vi "Add Timestamps to Rx Channels.vi"(8 "error in":errorcluster, 9 "timestamps":T1[](array[typedef]) format="%.0x", 10 "RxBC channel handles":T1[](array[typedef]) format="%.0x", 11 "RxRT channel handles":T1[](array[typedef]) format="%.0x") -> (0 "error out":errorcluster, 3 "Rx channel handles":T1[](array[typedef]) format="%.0x")   [LabVIEW 2020, in "Ballard MIL-STD-1553 Engine.lvlib" / "Implementation.lvlib" / "Execution Unit.lvclass"]
uses:
  Execution Unit.lvclass
  <vilib>/NI VeriStand/Custom Device API/Custom Device Item Ref.ctl
  <vilib>/NI VeriStand/Custom Device API/Custom Device API.lvlib
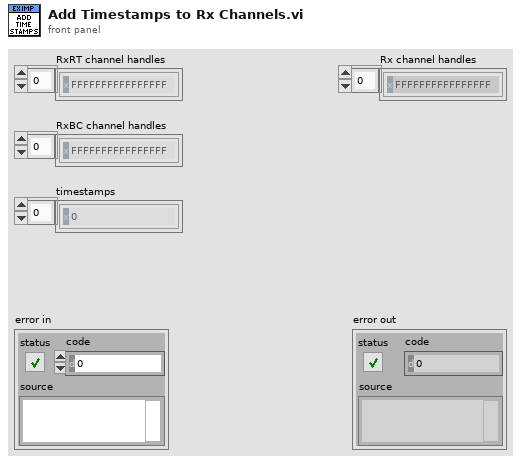
[diagram p1: front panel]
types:
  T1 = typedef "Custom Device API.lvlib/Custom Device Item Ref.ctl" = u64
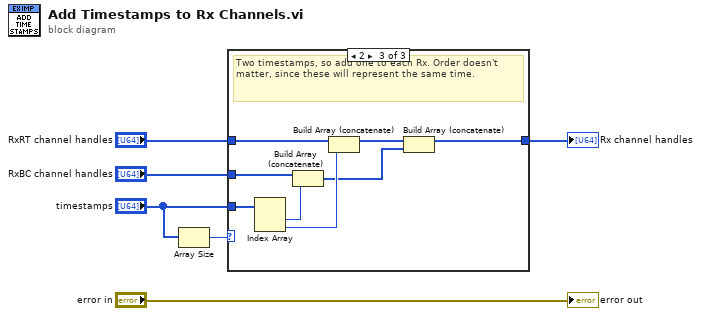
[diagram p0: block diagram]
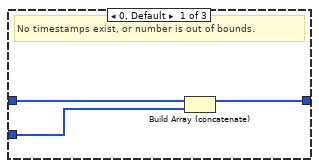
[diagram p2: hidden frame]
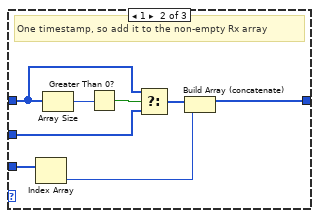
[diagram p3: hidden frame]
diagram:
  n1 = Array Size(array="timestamps") -> (size(s)=w5:i32)
  n2 = case shown="2" w5 {
    tunnel: "RxRT channel handles" -> [w9 w15 w22]
    tunnel: "RxBC channel handles" -> [w8 w14 w24]
    tunnel: [w7 w10 w18] -> w2
    tunnel: "timestamps" -> [_ w12 w25]
    frame 0, Default {
      # "No timestamps exist, or number is out of bounds."
      n3 = Build Array (concatenate)(w9, w8) -> (w7:T1[])
    }
    frame 1 {
      # "One timestamp, so add it to the non-empty Rx array"
      n4 = Index Array(array=w12) -> (element=w11:T1)  [unwired: 1 in]
      n5 = Array Size(array=w15) -> (size(s)=w17:i32)
      n6 = Greater Than 0?(x=w17) -> (x > 0?=w16:bool)
      n7 = Select(t=w15, s=w16, f=w14) -> (s? t:f=w13:T1[])
      n8 = Build Array (concatenate)(w13, w11) -> (w10:T1[])
    }
    frame 2 {
      # "Two timestamps, so add one to each Rx. Order doesn't matter, since these will represent the same time."
      n9 = Index Array(array=w25) -> (element #1=w23:T1, element #2=w21:T1)  [unwired: 2 in]
      n10 = Build Array (concatenate)(w24, w23) -> (w19:T1[])
      n11 = Build Array (concatenate)(w22, w21) -> (w20:T1[])
      n12 = Build Array (concatenate)(w20, w19) -> (w18:T1[])
    }
  }
  "Rx channel handles" <- w2
  "error out" <- "error in"
